vi "AES Decrypt (CBC).vi"(7 "Padding":i32(ring)=3 items=["None"=1, "PKCS7"=2, "Zeros"=3, "ANSIX923"=4, "ISO10126"=5], 8 "error in (no error)":errorcluster, 9 "IV":u8[](array[numeric]), 10 "Key":u8[](array[numeric]), 11 "Encrypted data in":u8[](array[numeric])) -> (0 "error out":errorcluster, 3 "Raw data out":u8[](array[numeric]))   [LabVIEW 2021, in "dotNET Crypto Symmetric Encryption.lvlib"]
doc: "Decrypt data using AES using the CBC cipher mode.\n\nThe Key, IV and padding mode must match the values used to encrypt the data."
uses:
  dotNET Crypto Symmetric Encryption.lvlib
  System.Core
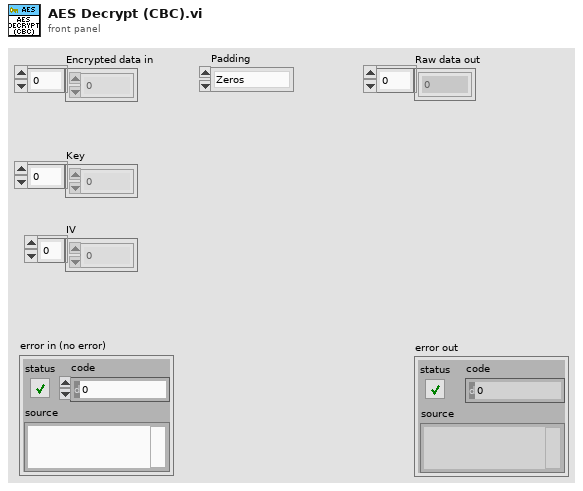
[diagram p1: front panel]
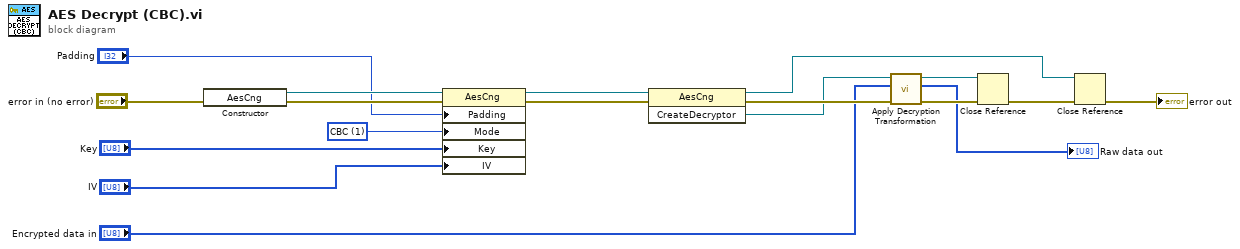
[diagram p0: block diagram]
diagram:
  w17 = 1 items=["CBC"=1, "ECB"=2, "OFB"=3, "CFB"=4, "CTS"=5] ("Mode")
  n1 = constructor class="AesCng"(error in="error in (no error)") -> (reference out=w13:refnum<k24>, error out=w14:errorcluster)  [unwired: 2 in, 1 out]
  n2 = property class="AesCng"(reference=w13, error in=w14, "Padding"="Padding", "Mode"=w17, "Key"="Key", "IV"="IV") -> (reference out=w15:refnum<k24>, error out=w16:errorcluster)
  n3 = invoke class="AesCng" method="CreateDecryptor"(reference=w15, error in=w16) -> (reference out=w10:refnum<k24>, error out=w8:errorcluster, "CreateDecryptor"=w5:refnum<k24>)  [unwired: 1 in]
  n4 = call "Apply Decryption Transformation.vi"("error in (no error)"=w8, "Encrypted data in"="Encrypted data in", "Crypto transform in"=w5) -> ("error out"=w7:errorcluster, "Plaintext"=→"Raw data out":u8[], "Crypto transform out"=w6:refnum<k24>)  [unwired: 6 in]
  n5 = Close Reference(reference=w6, error in (no error)=w7) -> (error out=w9:errorcluster)
  n6 = Close Reference(reference=w10, error in (no error)=w9) -> (error out=→"error out":errorcluster)
